vi "Init.vi"(8 "error in":errorcluster, 10 "Sourcegrid Container":refnum<k24>(container), 11 "MyEventGrid in":refnum<class "MyEventGrid.lvclass">) -> (0 "error out":errorcluster, 3 "MyEventGrid out":refnum<class "MyEventGrid.lvclass">)   [LabVIEW 2024, in "MyEventGrid.lvclass"]
uses:
  MyEventGrid.lvclass
  D:/git/Sourcegrid-LabVIEW/source/Grid/SourceGrid.lvclass
  source/Cells/Cell/Cell.lvclass
  source/Controllers/Custom Events/Custom Events.lvclass
  MyEventGrid.lvclass/MyEventGrid.ctl
  source/Grid/Set Column Default Width.vi
  source/Cells/Cell/Add Controller.vi
  source/Grid/SourceGrid.lvclass
  source/Editors/Combo Box/Combo Box.lvclass
  D:/git/Sourcegrid-LabVIEW/tests/MyEventGrid/MyEventGrid.lvclass
  D:/git/Sourcegrid-LabVIEW/source/Editors/Editor Base/Editor Control Base.lvclass
  D:/git/Sourcegrid-LabVIEW/source/Editors/Combo Box/Combo Box.lvclass
  D:/git/Sourcegrid-LabVIEW/dll/SourceGrid.dll
  dll/SourceGrid.dll
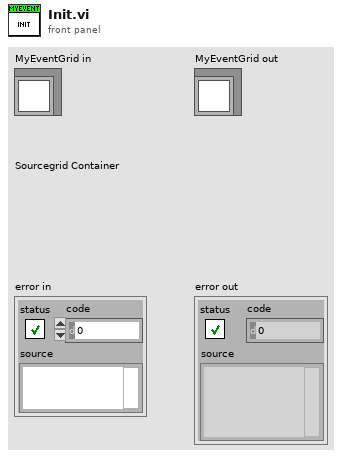
[diagram p1: front panel]
types:
  T1 = cluster{"onClick":refnum<user-event>, "onDoubleClick":refnum<user-event>, "onValueChanged":refnum<user-event>}
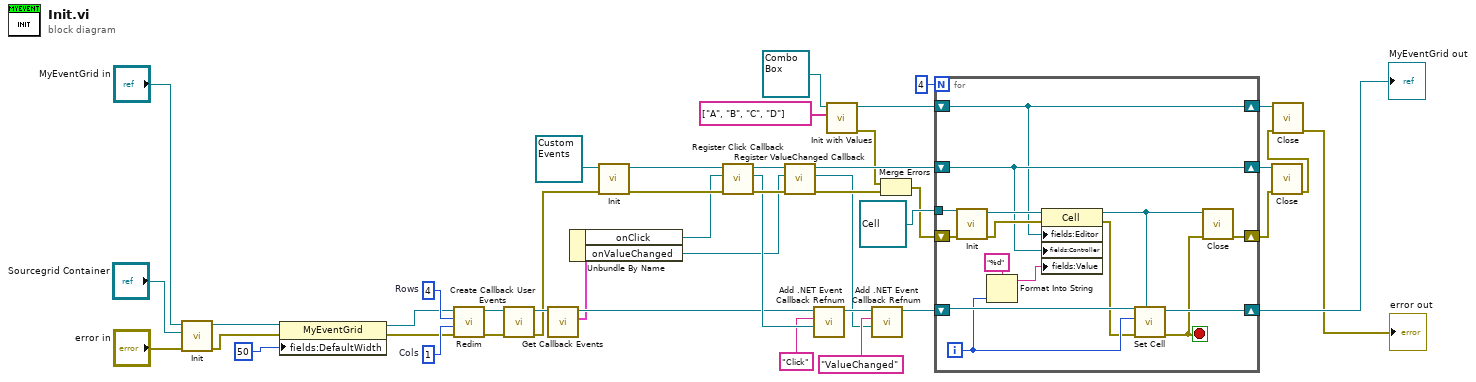
[diagram p0: block diagram]
diagram:
  w41 = 1  # Cols
  w42 = 4  # Rows
  n1 = call-parent "Init.vi"("error in"="error in", "Sourcegrid Container"="Sourcegrid Container", "Grid in"="MyEventGrid in") -> ("error out"=w33:errorcluster, "Grid out"=w32:refnum<class "MyEventGrid.lvclass">)  [unwired: 7 in]
  n2 = property class="MyEventGrid"(reference=w32, error in=w33, "fields:DefaultWidth"=50 ("DefaultWidth")) -> (reference out=w34:refnum<class "MyEventGrid.lvclass">, error out=w40:errorcluster)
  n3 = call "Redim.vi"("error in"=w40, "Columns"=w41, "Rows"=w42, "Sourcegrid in"=w34) -> ("error out"=w36:errorcluster, "Sourcegrid out"=w21:refnum<class "MyEventGrid.lvclass">)  [unwired: 6 in]
  n4 = call-dynamic "Create Callback User Events.vi"("error in"=w36, "MyEventGrid in"=w21) -> ("error out"=w16:errorcluster, "MyEventGrid out"=w20:refnum<class "MyEventGrid.lvclass">)  [unwired: 8 in]
  n5 = call "Get Callback Events.vi"("MyEventGrid in"=w20) -> ("Callback Events"=w18:T1, "MyEventGrid out"=w19:refnum<class "MyEventGrid.lvclass">)  [unwired: 9 in]
  n6 = Unbundle By Name(w18) -> ("onClick"=w17:refnum<user-event>, "onValueChanged"=w12:refnum<user-event>)
  n7 = call-dynamic "Init.vi"("error in"=w16, "Custom Events in"=refnum<class "Custom Events.lvclass"> refnum ("SourceGrid.lvlib:Custom Events.lvclass")) -> ("error out"=w27:errorcluster, "Custom Events out"=w25:refnum<class "Custom Events.lvclass">)  [unwired: 8 in]
  n8 = call-dynamic "Register Click Callback.vi"("error in"=w27, "onClick"=w17, "Custom Events in"=w25) -> ("error out"=w26:errorcluster, "Event Callback Refnum"=w24:refnum<k27>, "Custom Events out"=w14:refnum<class "Custom Events.lvclass">)  [unwired: 6 in]
  n9 = call-dynamic "Register ValueChanged Callback.vi"("error in"=w26, "onValueChanged"=w12, "Custom Events in"=w14) -> ("error out"=w15:errorcluster, "Event Callback Refnum"=w9:refnum<k27>, "Custom Events out"=w13:refnum<class "Custom Events.lvclass">)  [unwired: 6 in]
  n10 = call-dynamic "Add .NET Event Callback Refnum.vi"("Event Callback Refnum"=w24, "Event Name"="Click" ("Event"), "MyEventGrid in"=w19) -> ("MyEventGrid out"=w22:refnum<class "MyEventGrid.lvclass">)  [unwired: 8 in]
  n11 = call-dynamic "Init with Values.vi"("Values"=string[] ["A", "B", "C", "D"], "Combo Box in"=refnum<class "Combo Box.lvclass"> refnum ("SourceGrid.lvlib:Combo Box.lvclass")) -> ("error out"=w4:errorcluster, "Combo Box out"=w6:refnum<class "Combo Box.lvclass">)  [unwired: 8 in]
  n12 = call-dynamic "Add .NET Event Callback Refnum.vi"("Event Callback Refnum"=w9, "Event Name"="ValueChanged", "MyEventGrid in"=w22) -> ("MyEventGrid out"=w11:refnum<class "MyEventGrid.lvclass">)  [unwired: 8 in]
  n13 = Merge Errors(w4, w15) -> (w5:errorcluster)
  n14 = for {
    N: 4 -> [_]
    shift-right: [w49] -> w28
    shift-left: w5 -> [w50]
    shift-right: [w59] -> w30
    shift-left: w11 -> [w58]
    tunnel: refnum<class "Cell.lvclass"> refnum ("Cell in") -> [w54]
    shift-right: [w46] -> w29
    shift-left: w13 -> [w46]
    shift-right: [w45] -> w3
    shift-left: w6 -> [w45]
    i -> [w56]
    stop <- w51 stop-if-true
    n15 = call-dynamic "Init.vi"("error in"=w50, "Cell in"=w54) -> ("error out"=w52:errorcluster, "Cell out"=w53:refnum<class "Cell.lvclass">)  [unwired: 8 in]
    n16 = Format Into String(format string="%d", w56) -> (resulting string=w47:string)  [unwired: 2 in, 1 out]
    n17 = property class="Cell"(reference=w53, error in=w52, "fields:Editor"=w45, "fields:Controller"=w46, "fields:Value"=w47) -> (reference out=w48:refnum<class "Cell.lvclass">, error out=w55:errorcluster)
    n18 = call "Set Cell.vi"("Cell"=w48, "error in"=w55, "Row"=w56, "Sourcegrid in"=w58) -> ("error out"=w51:errorcluster, "Sourcegrid out"=w59:refnum<class "MyEventGrid.lvclass">)  [unwired: 6 in]
    n19 = call-dynamic "Close.vi"("error in"=w51, "Cell in"=w48) -> ("error out"=w49:errorcluster)  [unwired: 8 in, 1 out]
  }
  "MyEventGrid out" <- w30
  n20 = call-dynamic "Close.vi"("error in"=w28, "Custom Events in"=w29) -> ("error out"=w2:errorcluster)  [unwired: 8 in, 1 out]
  n21 = call-dynamic "Close.vi"("error in"=w2, "Combo Box in"=w3) -> ("error out"=→"error out":errorcluster)  [unwired: 8 in, 1 out]
